vi "setInputEnable.vi"(2 "enable":u32, 3 "ID":i32, 4 "handle":i32, 5 "错误输入（无错误）":errorcluster) -> (0 "return":i32, 1 "错误输出":errorcluster)   [LabVIEW 2013, in "EM_CVx.lvlib"]
uses:
  EM_CVx.lvlib
  library/moverLibrary_x86.dll
  library/moverLibrary_x64.dll
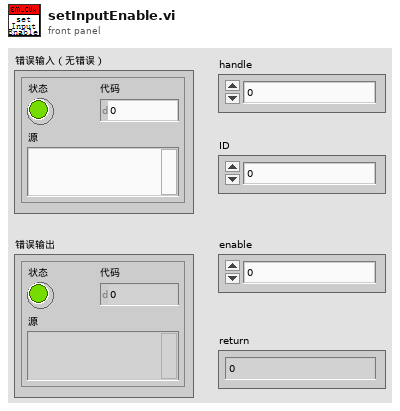
[diagram p1: front panel]
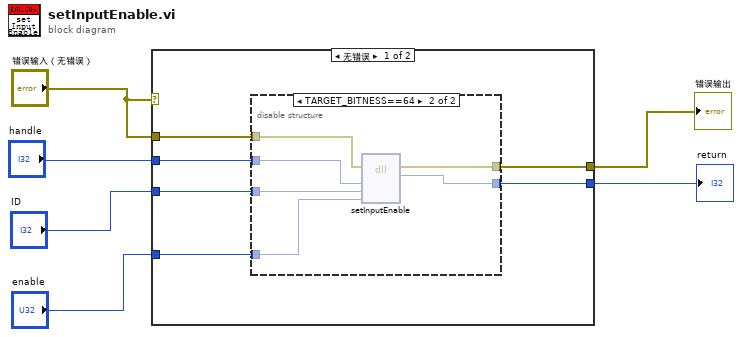
[diagram p0: block diagram]
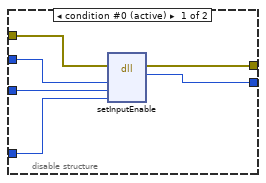
[diagram p2: hidden frame]
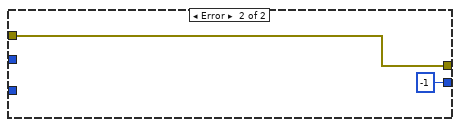
[diagram p3: hidden frame]
diagram:
  n1 = case shown="无错误" "错误输入（无错误）" {
    tunnel: "handle" -> [w12 _]
    tunnel: "ID" -> [w11 _]
    tunnel: "错误输入（无错误）" -> [w10 w26]
    tunnel: [w9 -1 ("return")] -> w4
    tunnel: [w8 w26] -> w3
    tunnel: "enable" -> [w7 _]
    frame No Error {
      n2 = disable-structure shown="TARGET_BITNESS==64" {
        disable-tunnel: w12 -> [w18 w22]
        disable-tunnel: w11 -> [w17 w23]
        disable-tunnel: w10 -> [w16 w21]
        disable-tunnel: [w15 w24] -> w9
        disable-tunnel: [w14 w20] -> w8
        disable-tunnel: w7 -> [w13 w19]
        frame condition #0 (active) {
          n3 = dll-call lib="E:/5-mover/4-labView/EM_CVx_2013/library/moverLibrary_x86.dll" fn="setInputEnable"(error in=w16, "handle"=w18, "ID"=w17, "enable"=w13) -> (error out=w14:errorcluster, "return"=w15:i32)  [unwired: 5 in, 1 out]
        }
        frame condition #1 {
          n4 = dll-call lib="E:/5-mover/4-labView/EM_CVx_2013/library/moverLibrary_x64.dll" fn="setInputEnable"(error in=w21, "handle"=w22, "ID"=w23, "enable"=w19) -> (error out=w20:errorcluster, "return"=w24:i32)  [unwired: 5 in, 1 out]
        }
      }
    }
    frame Error {
    }
  }
  "错误输出" <- w3
  "return" <- w4
